vi "texture.vi"(8 "Error In":errorcluster, 11 "QBrush In":refnum<class "QBrush.lvclass">) -> (0 "Error Out":errorcluster, 2 "Value":refnum<class "QPixmap.lvclass">, 3 "QBrush Out":refnum<class "QBrush.lvclass">)   [LabVIEW 2014, in "QBrush.lvclass"]
doc: "LabVIEW-specific documentation is not yet available. See <b>https://doc.qt.io/qt-5/qbrush.html#texture</b>"
uses:
  QBrush.lvclass
  QPixmap/QPixmap.lvclass
  LQ Core/LQSerialData/LQSerialData.lvclass/LQSerialData.ctl
  LQ Core/LQ Core.lvlib
  LQ Core/LQSerialData/LQSerialData.lvclass
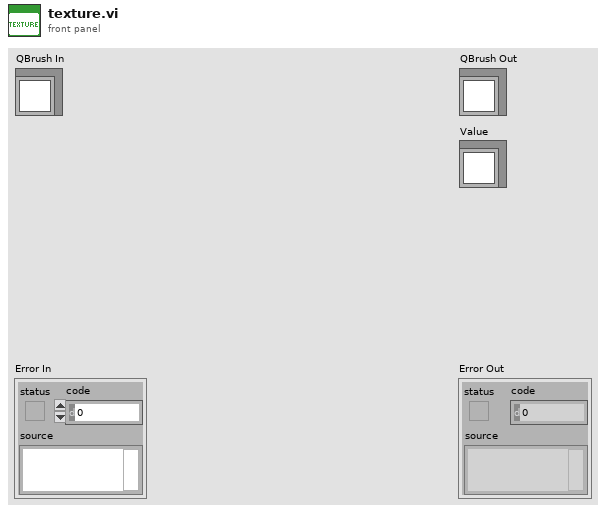
[diagram p1: front panel]
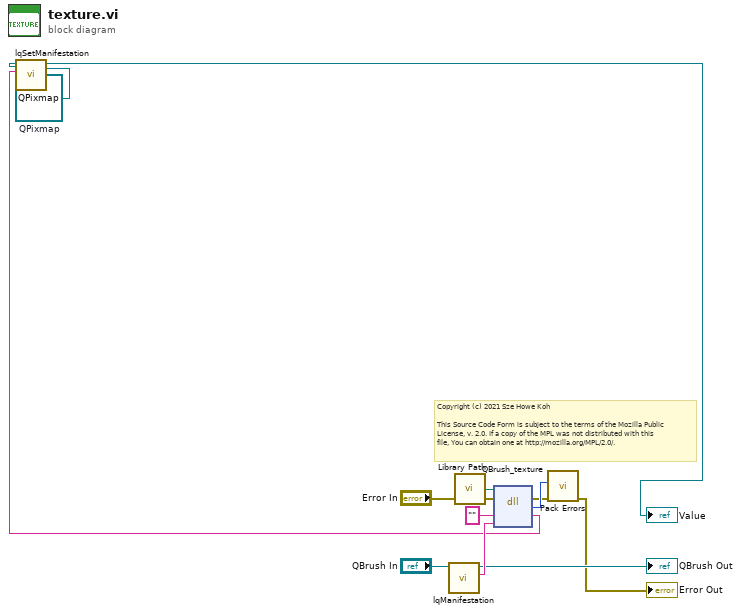
[diagram p0: block diagram]
diagram:
  w1 = refnum<class "QPixmap.lvclass"> refnum  # QPixmap
  # "Copyright (c) 2021 Sze Howe Koh\n\nThis Source Code Form is subject to the terms of the Mozilla Public\nLicense, v. 2.0. If a copy of the MPL was not distributed with this\nfile, You can obtain one at http://mozilla.org/MPL/2.0/."
  n1 = call "lqManifestation.vi"("LQSerialData in"="QBrush In") -> ("Manifestation"=w10:string, "LQSerialData out"=→"QBrush Out":refnum<class "QBrush.lvclass">)  [unwired: 9 in]
  n2 = call "Library Path.vi"() -> ("Library Path"=w7:path)
  n3 = dll-call lib="?" fn="QBrush_texture"(path in=w7, error in="Error In", "_retVal"="" ("retVal"), "_instance"=w10) -> (error out=w5:errorcluster, w6:i32, "_retVal"=w2:string)  [unwired: 2 in, 1 out]
  n4 = call "lqSetManifestation.vi"("Manifestation"=w2, "LQSerialData in"=w1) -> ("LQSerialData out"=→"Value":refnum<class "QPixmap.lvclass">)  [unwired: 8 in, 1 out]
  n5 = call "Pack Errors.vi"("Error In"=w5, "Error Code"=w6) -> ("Error Out"=→"Error Out":errorcluster)  [unwired: 9 in]
